vi "RSZVB Configure External Generator.vi"(0 "VISA session":refnum<visa-resource-name>, 1 "Interface Address":string, 2 "10 MHz Reference Frequency (F: Off)":bool, 5 "Generator Number (1)":i32=1, 7 "Generator Name":string, 9 "Generator Type":string, 11 "error in (no error)":errorcluster {"code" format="%.0x"}, 12 "Fast Sweep Mode (F: Off)":bool, 13 "Interface Type":string) -> (4 "dup VISA session":refnum<visa-resource-name>, 15 "error out":errorcluster {"code" format="%.0x"})   [LabVIEW 2011]
doc: "This VI configures an external generator and adds it to the list of available generators.\n\nRemote-control command(s):\nSYSTem:COMMunicate:RDEVice:GENerator<gen_no>:DEFine\n'<gen_name>', '<driver>', '<interface>', '<address>'[, <fast_sweep>, <10_MHz_Ref>]"
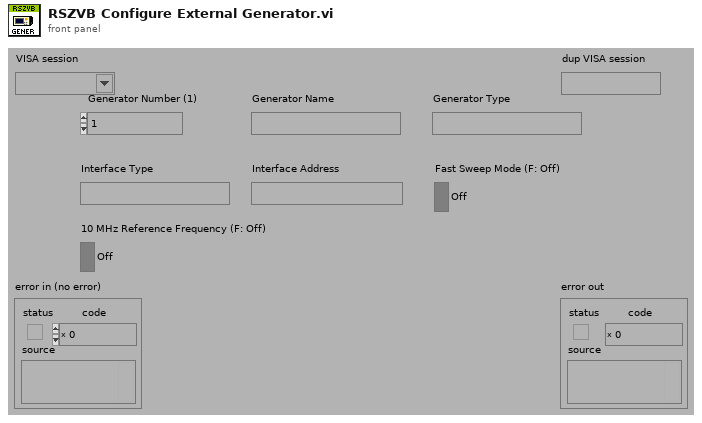
[diagram p1: front panel]
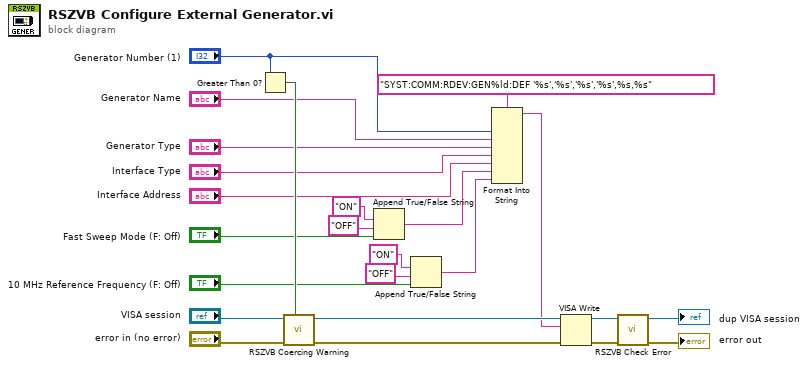
[diagram p0: block diagram]
diagram:
  n1 = Greater Than 0?(x="Generator Number (1)") -> (x > 0?=w18:bool)
  n2 = call "RSZVB Coercing Warning.vi"("In Range?"=w18, "error in (no error)"="error in (no error)", "VISA session"="VISA session") -> ("error out"=w23:errorcluster, "dup VISA session"=w24:refnum<visa-resource-name>)  [unwired: 7 in]
  n3 = Append True/False String(1:"Fast Sweep Mode (F: Off)", 2:"OFF", 3:"ON") -> (0:w3:string)  [unwired: 1 in]
  n4 = Append True/False String(1:"10 MHz Reference Frequency (F: Off)", 2:"OFF", 3:"ON") -> (0:w2:string)  [unwired: 1 in]
  n5 = Format Into String(format string="SYST:COMM:RDEV:GEN%ld:DEF '%s','%s','%s','%s',%s,%s", "Generator Number (1)", "Generator Name", "Generator Type", "Interface Type", "Interface Address", w3, w2) -> (resulting string=w1:string)  [unwired: 2 in, 1 out]
  n6 = VISA Write(VISA resource name=w24, write buffer=w1, error in (no error)=w23) -> (VISA resource name out=w21:refnum<visa-resource-name>, error out=w22:errorcluster)  [unwired: 1 out]
  n7 = call "RSZVB Check Error.vi"("error in (no error)"=w22, "VISA session"=w21) -> ("error out"=→"error out":errorcluster, "dup VISA session"=→"dup VISA session":refnum<visa-resource-name>)  [unwired: 8 in]
